vi "run_chatcompletion_core.vi"(0 "chatcompletion_llm_interface in":refnum<class "llm_openai_chatmodels.lvclass">, 5 "Messages":refnum<class "abstract_message_base.lvclass">[](array[class]), 11 "error in (no error)":errorcluster) -> (4 "chatcompletion_llm_interface out":refnum<class "llm_openai_chatmodels.lvclass">, 6 "Response":refnum<class "abstract_message_base.lvclass">, 15 "error out":errorcluster)   [LabVIEW 2020, in "llm_openai_chatmodels.lvclass"]
uses:
  llm_openai_chatmodels.lvclass
  abstract_message_base/abstract_message_base.lvclass
  message_text/message_text.lvclass
  D:/Personal/LabVIEW LLMs/src/models/abstract_message_base/abstract_message_base.lvclass
  message_text/message.ctl
  <vilib>/httpClient/POSTBuffer.vi
  llm_openai_chatmodels.lvclass/llm_openai_chatmodels.ctl
  <vilib>/httpClient/LabVIEWHTTPClient.lvlib
panel:
  out "body":string
  out "headers":string
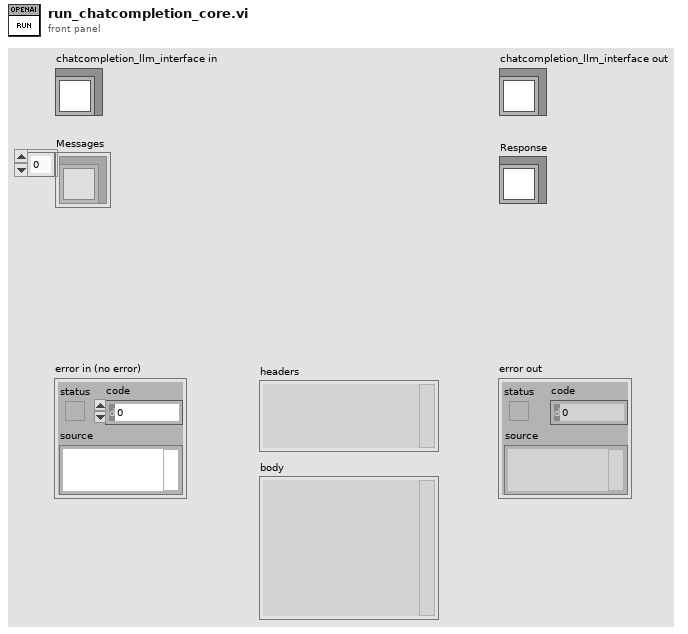
[diagram p1: front panel]
types:
  T1 = typedef "message_text.lvclass/message.ctl" = cluster{"role":string, "content":string[]}
  T2 = typedef "LabVIEWHTTPClient.lvlib/ClientHandle.ctl" = refnum<k1>
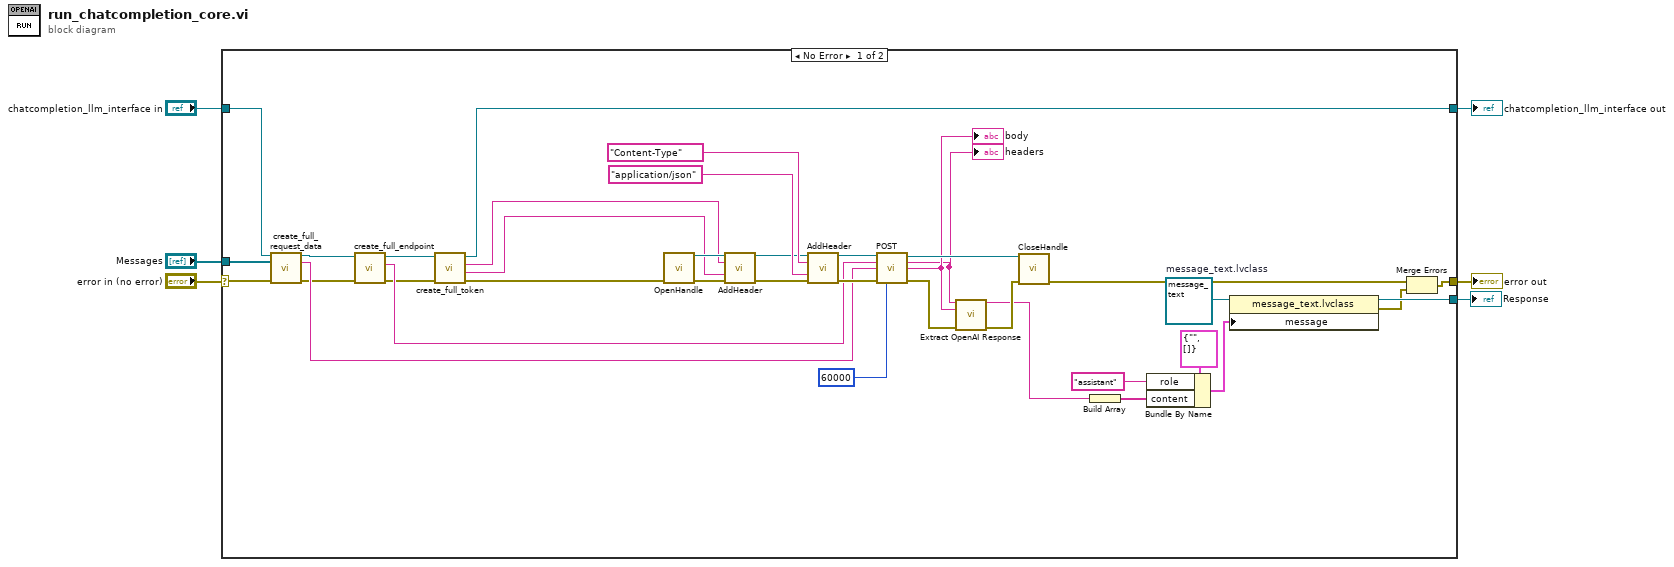
[diagram p0: block diagram]
diagram:
  n1 = case shown="No Error" "error in (no error)" {
    selector: "error in (no error)" -> [w26 w45]
    tunnel: [w29 w45] -> w5
    tunnel: "chatcompletion_llm_interface in" -> [w28 w44]
    tunnel: [w18 w44] -> w3
    tunnel: "Messages" -> [w27 _]
    tunnel: [w8 _] -> w1
    frame No Error {
      w14 = refnum<class "message_text.lvclass"> refnum  # message_text.lvclass
      n2 = call-dynamic "create_full_request_data.vi"("llm_openai_chatmodels in"=w28, "Messages"=w27, "error in (no error)"=w26) -> ("llm_openai_chatmodels out"=w24:refnum<class "llm_openai_chatmodels.lvclass">, "Request Data"=w25:string, "error out"=w23:errorcluster)  [unwired: 10 in]
      n3 = call-dynamic "create_full_endpoint.vi"("error in (no error)"=w23, "llm_openai_chatmodels in"=w24) -> ("error out"=w21:errorcluster, "endpoint"=w22:string, "llm_openai_chatmodels out"=w19:refnum<class "llm_openai_chatmodels.lvclass">)  [unwired: 7 in]
      n4 = call-dynamic "create_full_token.vi"("error in (no error)"=w21, "llm_openai_chatmodels in"=w19) -> ("error out"=w20:errorcluster, "token"=w16:string, "header"=w17:string, "llm_openai_chatmodels out"=w18:refnum<class "llm_openai_chatmodels.lvclass">)  [unwired: 6 in]
      n5 = call <vilib>:"OpenHandle.vi"("error in (no error)"=w20) -> ("client handle out"=w43:T2, "error out"=w42:errorcluster)  [unwired: 13 in]
      n6 = call <vilib>:"AddHeader.vi"("client handle"=w43, "header"=w17, "value"=w16, "error in (no error)"=w42) -> ("client handle out"=w39:T2, "error out"=w37:errorcluster)  [unwired: 10 in]
      n7 = call <vilib>:"AddHeader.vi"("client handle"=w39, "header"="Content-Type", "value"="application/json", "error in (no error)"=w37) -> ("client handle out"=w38:T2, "error out"=w36:errorcluster)  [unwired: 10 in]
      n8 = call-poly <vilib>:"POST.vi"("client handle"=w38, "url"=w22, "buffer"=w25, "error in (no error)"=w36, "timeout (10000)"=60000) -> ("client handle out"=w34:T2, "headers"=w30:string, "body"=w31:string, "error out"=w33:errorcluster)  [unwired: 7 in]
      "headers" <- w30
      "body" <- w31
      n9 = call "Extract OpenAI Response.vi"("headers"=w30, "body"=w31, "error in"=w33) -> ("value"=w10:string, "error out"=w32:errorcluster)  [unwired: 11 in]
      n10 = call <vilib>:"CloseHandle.vi"("client handle"=w34, "error in (no error)"=w32) -> ("error out"=w35:errorcluster)  [unwired: 13 in]
      n11 = Build Array(w10) -> (w11:string[])
      n12 = Bundle By Name(cluster=T1 {"role"="", "content"=[]} ("message"), "role"="assistant", "content"=w11) -> (w9:T1)
      n13 = property class="message_text.lvclass"(reference=w14, "message"=w9) -> (reference out=w8:refnum<class "message_text.lvclass">, error out=w7:errorcluster)  [unwired: 1 in]
      n14 = Merge Errors(w35, w7) -> (w29:errorcluster)
    }
    frame Error {
    }
  }
  "error out" <- w5
  "chatcompletion_llm_interface out" <- w3
  "Response" <- w1
